vi "Send Shutdown Message.vi"(8 "error in (no error)":errorcluster, 11 "msg cluster":T1) -> (0 "error out":errorcluster)   [LabVIEW 2020]
uses:
  Messaging Cluster.ctl
  Hardware/Sensors/Cameras/Camera.lvclass
  C:/Users/jharw/Documents/1 Folder to Rule them All/UMD/Inflation-Apparatus/src/Hardware/General Hardware.lvclass
  Hardware/Sensors/Force Sensors/Force Sensor.lvclass
  Hardware/Actuators/Servos/Servo.lvclass
  Hardware/Actuators/Switches/Switch.lvclass
  Controller Loop/Message and Data.ctl
  Inflation Test/Parameter Class/IA Test Parameters.lvclass
  Controllers/Controller.lvclass
  GUI/Main GUI Loop/Handler.ctl
  Inflation Test/Result Handling/Inflation Test Numeric Results.ctl
  Hardware/General Hardware.lvclass/General Hardware.ctl
  Hardware/General Hardware.lvclass
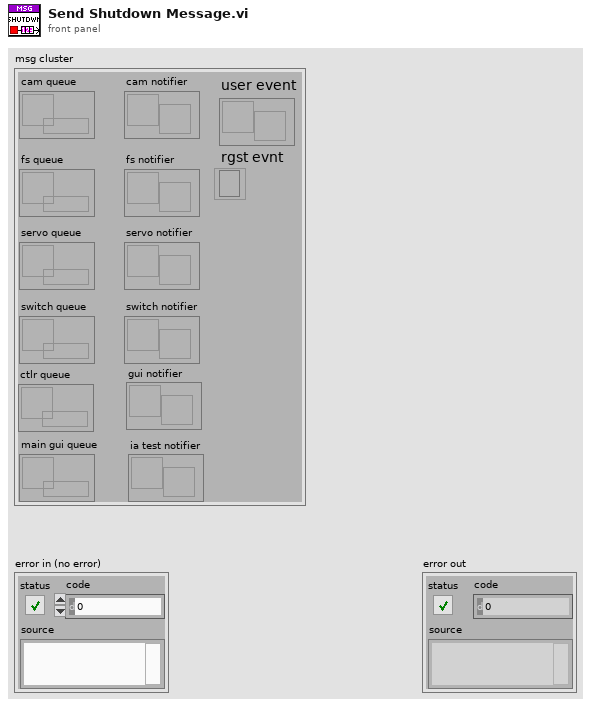
[diagram p1: front panel]
types:
  T1 = typedef "Messaging Cluster.ctl" = cluster{"cam queue":refnum<queue>, "fs queue":refnum<queue>, "servo queue":refnum<queue>, "switch queue":refnum<queue>, "switch notifier":refnum<notifier>, "servo notifier":refnum<notifier>, "fs notifier":refnum<notifier>, "cam notifier":refnum<notifier>, "rgst evnt":refnum<event-registration>, "user event":refnum<user-event>, "ctlr queue":refnum<queue>, "main gui queue":refnum<queue>, "gui notifier":refnum<notifier>, "ia test notifier":refnum<notifier>}
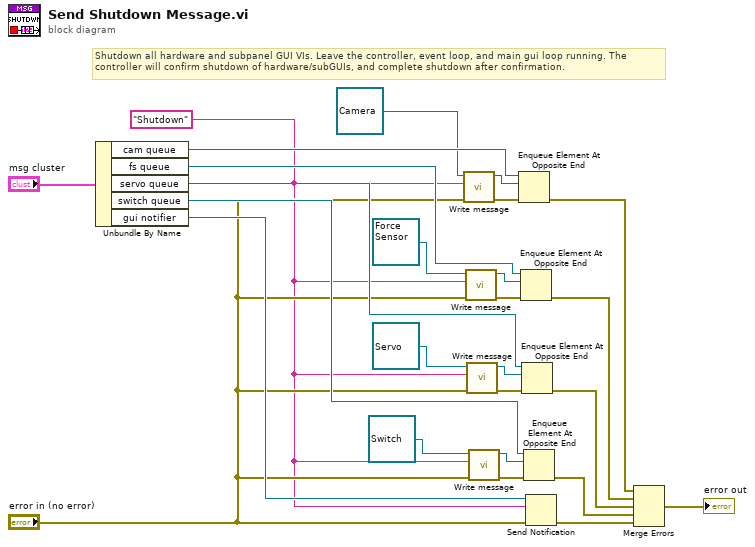
[diagram p0: block diagram]
diagram:
  w6 = "Shutdown"
  # "Shutdown all hardware and subpanel GUI VIs. Leave the controller, event loop, and main gui loop running. The controller will confirm shutdown of hardware/subGUIs, and complete shutdown after confirmation."
  n1 = Unbundle By Name("msg cluster") -> ("cam queue"=w24:refnum<queue>, "fs queue"=w18:refnum<queue>, "servo queue"=w15:refnum<queue>, "switch queue"=w14:refnum<queue>, "gui notifier"=w8:refnum<notifier>)
  n2 = call "Write message.vi"("error in (no error)"="error in (no error)", "message"=w6, "General Hardware in"=refnum<class "Camera.lvclass"> refnum ("Camera.lvclass")) -> ("error out"=w26:errorcluster, "General Hardware out"=w25:refnum<class "Camera.lvclass">)  [unwired: 7 in]
  n3 = call "Write message.vi"("error in (no error)"="error in (no error)", "message"=w6, "General Hardware in"=refnum<class "Force Sensor.lvclass"> refnum ("Force Sensor.lvclass")) -> ("error out"=w21:errorcluster, "General Hardware out"=w20:refnum<class "Force Sensor.lvclass">)  [unwired: 7 in]
  n4 = call "Write message.vi"("error in (no error)"="error in (no error)", "message"=w6, "General Hardware in"=refnum<class "Servo.lvclass"> refnum ("Servo.lvclass")) -> ("error out"=w22:errorcluster, "General Hardware out"=w19:refnum<class "Servo.lvclass">)  [unwired: 7 in]
  n5 = call "Write message.vi"("error in (no error)"="error in (no error)", "message"=w6, "General Hardware in"=refnum<class "Switch.lvclass"> refnum ("Switch.lvclass")) -> ("error out"=w16:errorcluster, "General Hardware out"=w17:refnum<class "Switch.lvclass">)  [unwired: 7 in]
  n6 = Enqueue Element At Opposite End(queue=w24, element=w25, error in (no error)=w26) -> (error out=w10:errorcluster)  [unwired: 1 in, 2 out]
  n7 = Enqueue Element At Opposite End(queue=w18, element=w20, error in (no error)=w21) -> (error out=w11:errorcluster)  [unwired: 1 in, 2 out]
  n8 = Enqueue Element At Opposite End(queue=w15, element=w19, error in (no error)=w22) -> (error out=w12:errorcluster)  [unwired: 1 in, 2 out]
  n9 = Enqueue Element At Opposite End(queue=w14, element=w17, error in (no error)=w16) -> (error out=w13:errorcluster)  [unwired: 1 in, 2 out]
  n10 = Send Notification(notification=w6, notifier=w8, error in (no error)="error in (no error)") -> (error out=w5:errorcluster)  [unwired: 1 out]
  n11 = Merge Errors(w10, w11, w12, w13, w5) -> (→"error out":errorcluster)
